vi "SingleConnection.vi"() -> ()   [LabVIEW 2013, in "WebSockets.lvlib"]
uses:
  WebSockets.lvlib
panel:
  in  "stop":bool
  out "Received Data":string
  in  "Send":bool
  in  "String":string
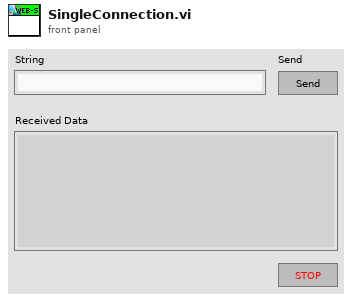
[diagram p1: front panel]
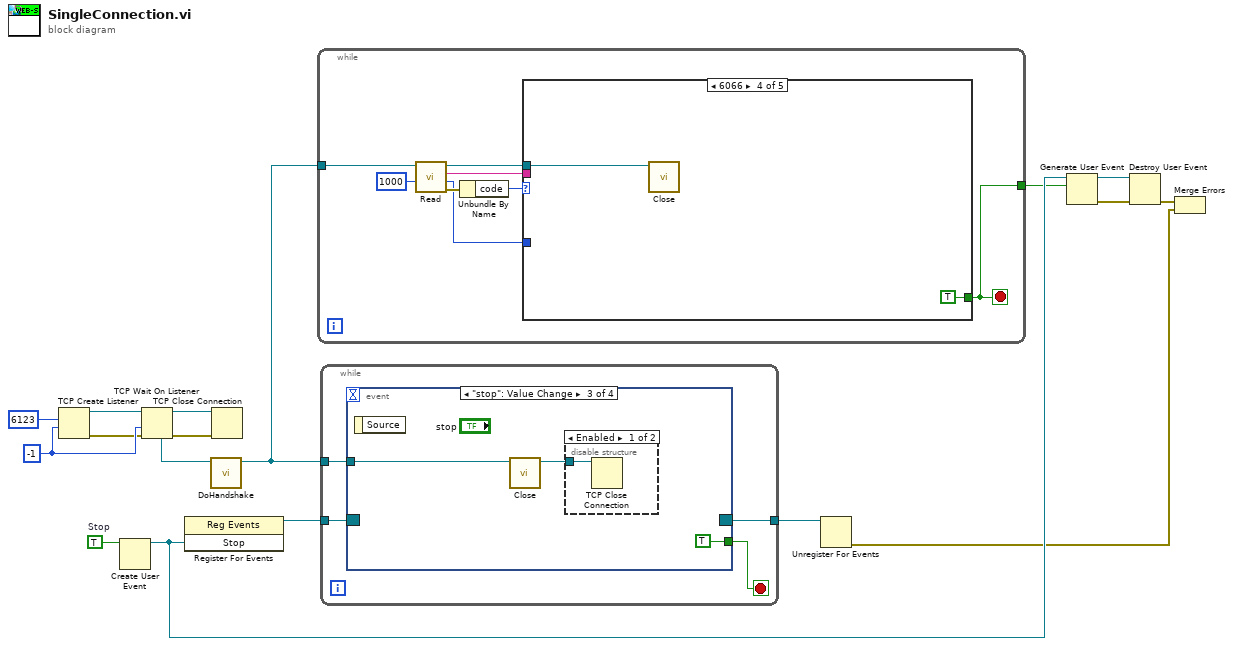
[diagram p0: block diagram]
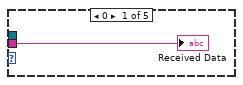
[diagram p2: hidden frame]
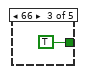
[diagram p4: hidden frame]
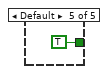
[diagram p5: hidden frame]
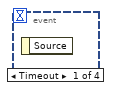
[diagram p6: hidden frame]
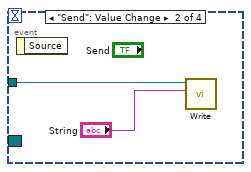
[diagram p7: hidden frame]
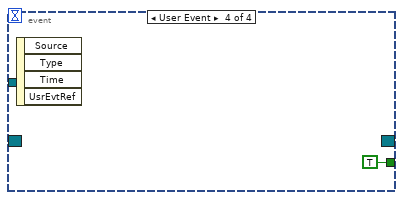
[diagram p9: hidden frame]
diagram:
  w8 = TRUE  # Stop
  w15 = -1 ("timeout ms (25000)")
  n1 = TCP Create Listener(9:w15, 10:u16 6123 ("port")) -> (0:w13:errorcluster, 3:w14:refnum<k5>)  [unwired: 3 in, 1 out]
  n2 = Create User Event(user event datatype=w8) -> (user event=w6:refnum<user-event>)  [unwired: 1 in, 1 out]
  n3 = TCP Wait On Listener(8:w13, 9:w15, 11:w14) -> (0:w10:errorcluster, 3:w11:refnum<k5>, 4:w12:refnum<k5>)  [unwired: 1 in, 2 out]
  n4 = register-events(w6) -> (reference out=w9:refnum<event-registration>)  [unwired: 2 in, 1 out]
  n5 = call "DoHandshake.vi"("TCP Network Connection in"=w12) -> ("TCP Network Connection out"=w17:refnum<k5>)  [unwired: 8 in, 2 out]
  n6 = TCP Close Connection(connection ID=w11, error in (no error)=w10) -> ()  [unwired: 1 in, 2 out]
  n7 = while {
    tunnel: w17 -> [w25]
    tunnel: [w20] -> w5
    stop <- w20 stop-if-true
    n8 = call "Read.vi"("timeout ms (25000)"=1000, "connection ID"=w25) -> ("error out"=w23:errorcluster, "Opcode"=w18:u8, "Data"=w21:string, "connection ID out"=w19:refnum<k5>)  [unwired: 6 in]
    n9 = Unbundle By Name(w23) -> ("code"=w22:i32)
    n10 = case shown="6066" w22 {
      tunnel: w21 -> [w26 _ _ _ _]
      tunnel: [_ _ TRUE TRUE TRUE] -> w20
      tunnel: w19 -> [_ _ _ w29 _]
      tunnel: w18 -> [_ _ _ _ _]
      frame 0 {
        "Received Data" <- w26
      }
      frame 56 {
      }
      frame 66 {
      }
      frame 6066 {
        n11 = call "Close.vi"("connection ID"=w29) -> ()  [unwired: 9 in, 2 out]
      }
      frame Default {
      }
    }
  }
  n12 = while {
    tunnel: w17 -> [w34]
    tunnel: w9 -> [w32]
    tunnel: [w31] -> w7
    stop <- w33 stop-if-true
    n13 = event shown="[2] \"stop\": Value Change" {
      selector: w32 -> [_ _ _ _]
      dyn-events: [_ _ _ _] -> w31
      timeout: _ -> [_ _ _ _]
      tunnel: w34 -> [_ w36 w38 _]
      tunnel: [_ _ TRUE TRUE] -> w33
      event Timeout {
        n14 = event-data() -> ()  [unwired: 1 in, 1 out]
      }
      event "Send": Value Change {
        n15 = event-data() -> ()  [unwired: 1 in, 1 out]
        n16 = call "Write.vi"("Data"="String", "connection ID"=w36) -> ()  [unwired: 8 in, 2 out]
      }
      event "stop": Value Change {
        n17 = event-data() -> ()  [unwired: 1 in, 1 out]
        n18 = call "Close.vi"("connection ID"=w38) -> ("connection ID out"=w37:refnum<k5>)  [unwired: 9 in, 1 out]
        n19 = disable-structure shown="Enabled" {
          disable-tunnel: w37 -> [w40 _]
          frame Enabled {
            n20 = TCP Close Connection(connection ID=w40) -> ()  [unwired: 2 in, 2 out]
          }
          frame Disabled {
          }
        }
      }
      event User Event {
        n21 = event-data() -> ()  [unwired: 1 in, 4 out]
      }
    }
  }
  n22 = Unregister For Events(event registration refnum=w7) -> (error out=w1:errorcluster)  [unwired: 1 in]
  n23 = Generate User Event(user event=w6, event data cluster=w5) -> (user event out=w4:refnum<user-event>, error out=w3:errorcluster)  [unwired: 2 in]
  n24 = Destroy User Event(user event=w4, error in=w3) -> (error out=w2:errorcluster)
  n25 = Merge Errors(w2, w1) -> ()  [unwired: 1 out]
